vi "Execute.vi"(5 "SleepTerminalArray":refnum<vi>, 6 "ExeRef":refnum<vi>, 7 "ActiveTerminalArray":refnum<vi>, 8 "error in (no error)":errorcluster, 9 "Json_In":string, 10 "VariableRef":T2, 11 "Info":T1) -> (0 "Error Out":errorcluster, 1 "NumResultArray":dbl[](array[numeric]), 2 "StrResultArray":string[](array[string]), 3 "StrResult":string, 4 "NumResult":dbl)   [LabVIEW 2018, in "Array.lvlib"]
uses:
  Array.lvlib
  <userlib>/_OpenG.lib/dictionary/dictionary.llb/Dictionary Object RefNum__ogtk.ctl
  <userlib>/_OpenG.lib/dictionary/dictionary.llb/Dictionary Object RefNum - Enum__ogtk.ctl
  <userlib>/_MGI/1D Array/MGI Average/MGI Average (DBL[]).vi
  <userlib>/_OpenG.lib/array/array.llb/Remove Duplicates from 1D Array (String)__ogtk.vi
  <vilib>/addons/_JKI.lib/Serialization/JSON/JKI JSON Serialization.lvlib
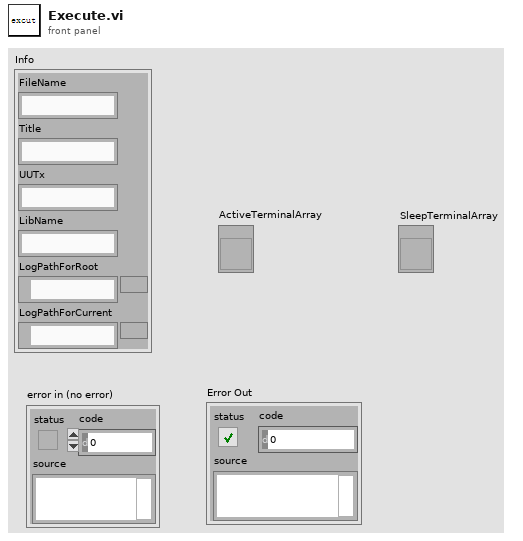
[diagram p1: front panel]
types:
  T1 = cluster{"FileName":string, "Title":string, "UUTx":string, "LibName":string, "LogPathForRoot":path, "LogPathForCurrent":path}
  T2 = typedef "Dictionary Object RefNum__ogtk.ctl" = refnum<k1>
  T3 = cluster{"ArraySize":cluster{"json":cluster{"Method":string, "ArrayVar":string}}, "IndexArray":cluster{"json":cluster{"Method":string, "ArrayVar":string, "Index":i32}}, "BuildArray":cluster{"json":cluster{"Method":string, "FirstElementVar":string, "SecondElementVar":string}}, "InsertIntoArray":cluster{"json":cluster{"Method":string, "ArrayVar":string, "Index":i32, "SubArrayVar":string}}, "DeleteFromArray":cluster{"json":cluster{"Method":string, "ArrayVar":string, "Index":i32, "Length":i32}}, "InitializeArray":cluster{"json":cluster{"Method":string, "ElementVar":string, "DimensionSize":i32}}, "ArraySubset":cluster{"json":cluster{"Method":string, "ArrayVar":string, "Index":i32, "Length":i32}}, "ArrayMax":cluster{"json":cluster{"Method":string, "ArrayVar":string}}, "ArrayMin":cluster{"json":cluster{"Method":string, "ArrayVar":string}}, "SearchArray":cluster{"json":cluster{"Method":string, "ArrayVar":string, "ElementVar":string, "StartIndex":i32}}, "ReplaceArraySubset":cluster{"json":cluster{"Method":string, "ArrayVar":string, "Index":i32, "SubArrayVar":string}}, "SortArray":cluster{"json":cluster{"Method":string, "ArrayVar":string}}, "ReverseArray":cluster{"json":cluster{"Method":string, "ArrayVar":string}}, "ArrayAverage":cluster{"json":cluster{"Method":string, "NumArrayVar":string, "IgnoreNaN":bool}}, "RemoveDuplicatesFromArray":cluster{"json":cluster{"Method":string, "ArrayVar":string}}, "ArrayToString":cluster{"json":cluster{"Method":string, "ArrayVar":string, "Delimiter":string}}}
  T4 = cluster{"json":cluster{"Method":string, "ArrayVar":string}}
  T5 = cluster{"json":cluster{"Method":string, "ArrayVar":string, "Index":i32}}
  T6 = cluster{"json":cluster{"Method":string, "FirstElementVar":string, "SecondElementVar":string}}
  T7 = cluster{"json":cluster{"Method":string, "ArrayVar":string, "Index":i32, "SubArrayVar":string}}
  T8 = cluster{"json":cluster{"Method":string, "ArrayVar":string, "Index":i32, "Length":i32}}
  T9 = cluster{"json":cluster{"Method":string, "ElementVar":string, "DimensionSize":i32}}
  T10 = cluster{"json":cluster{"Method":string, "ArrayVar":string, "ElementVar":string, "StartIndex":i32}}
  T11 = cluster{"json":cluster{"Method":string, "NumArrayVar":string, "IgnoreNaN":bool}}
  T12 = cluster{"json":cluster{"Method":string, "ArrayVar":string, "Delimiter":string}}
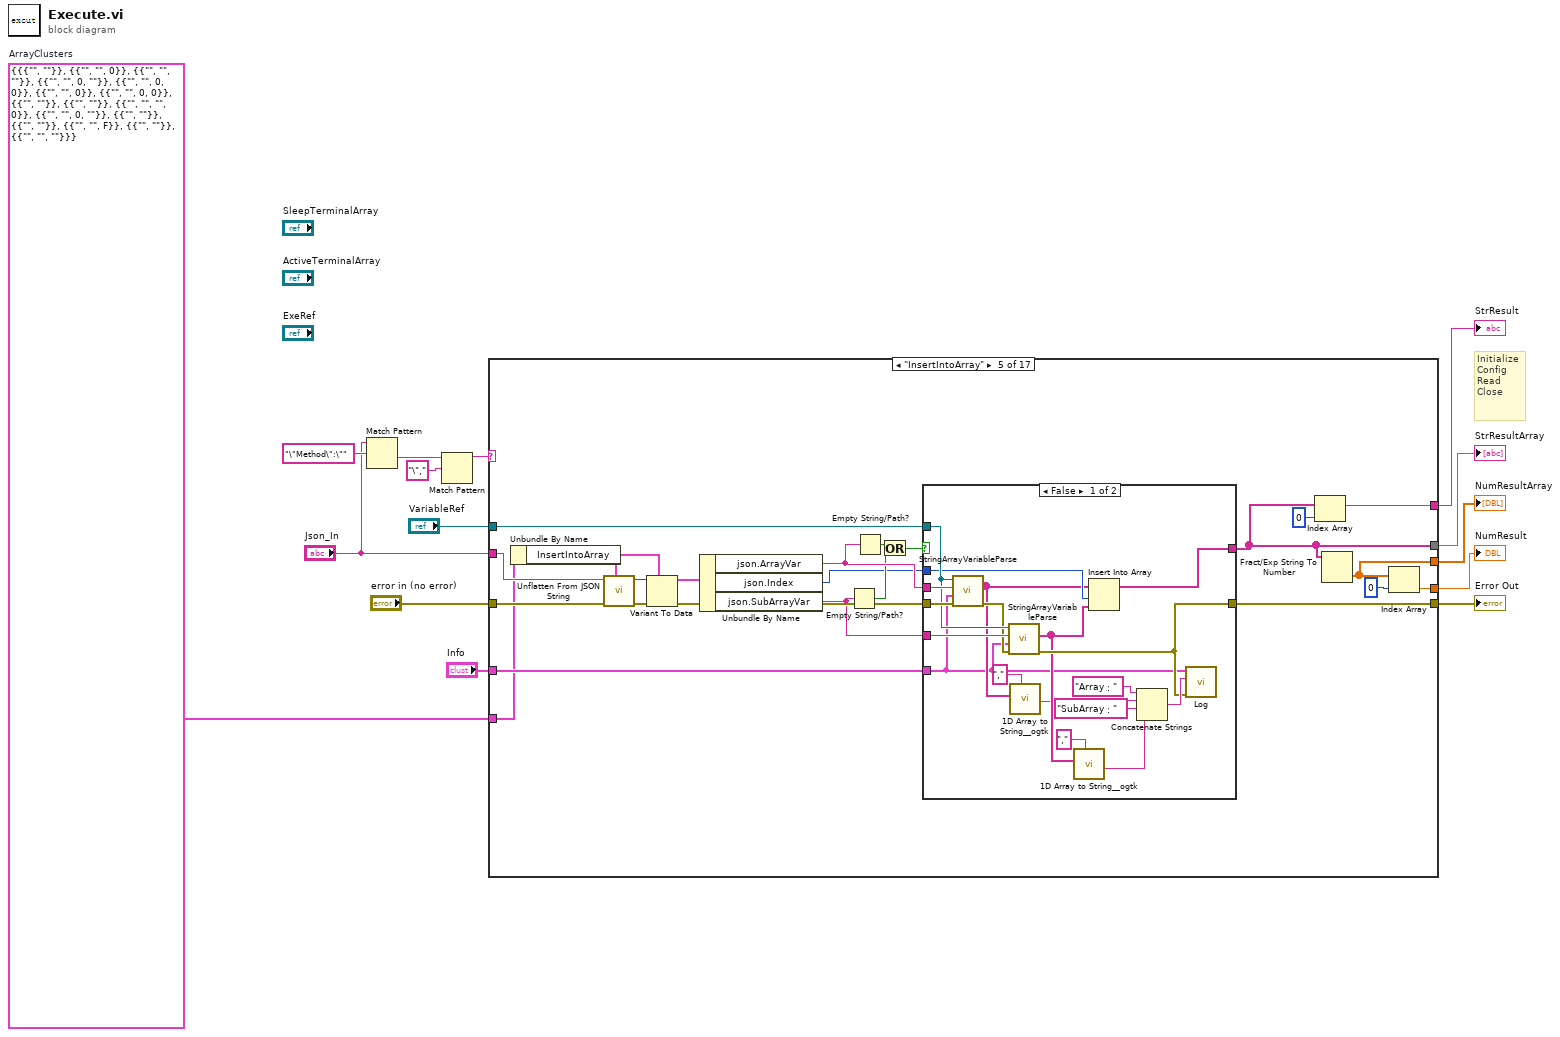
[diagram p0: block diagram]
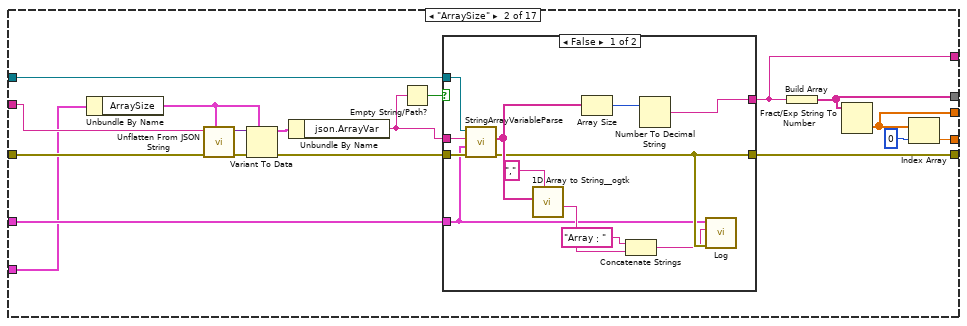
[diagram p3: hidden frame]
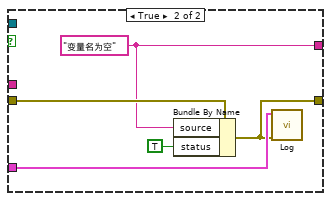
[diagram p4: hidden frame]
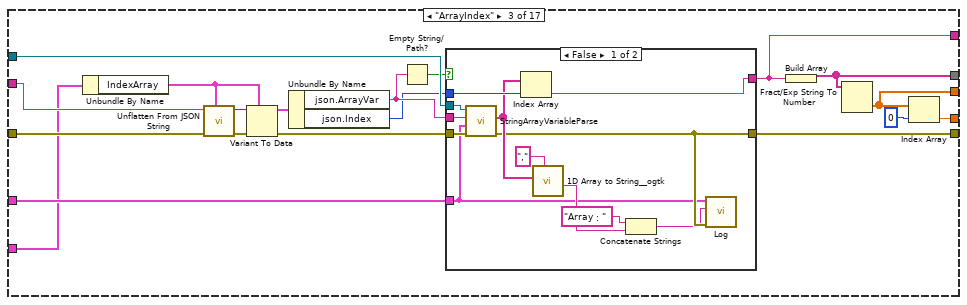
[diagram p5: hidden frame]
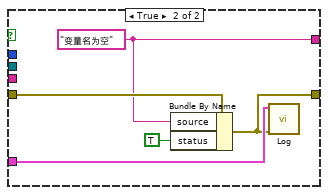
[diagram p6: hidden frame]
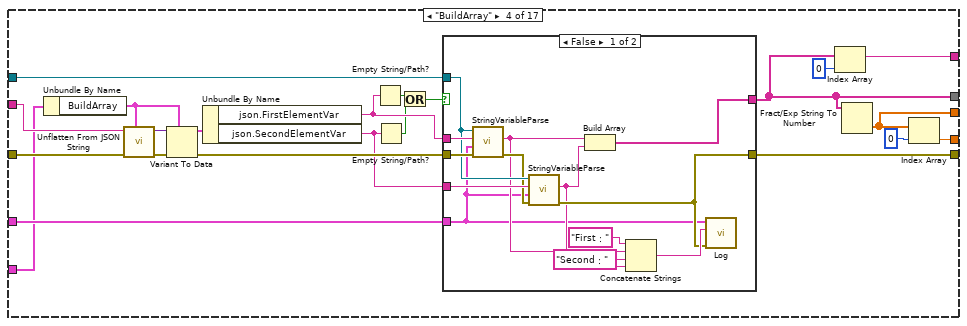
[diagram p7: hidden frame]
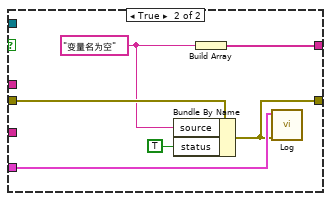
[diagram p8: hidden frame]
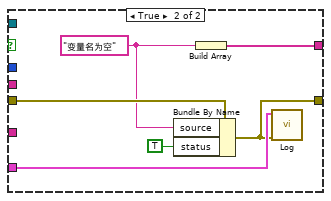
[diagram p9: hidden frame]
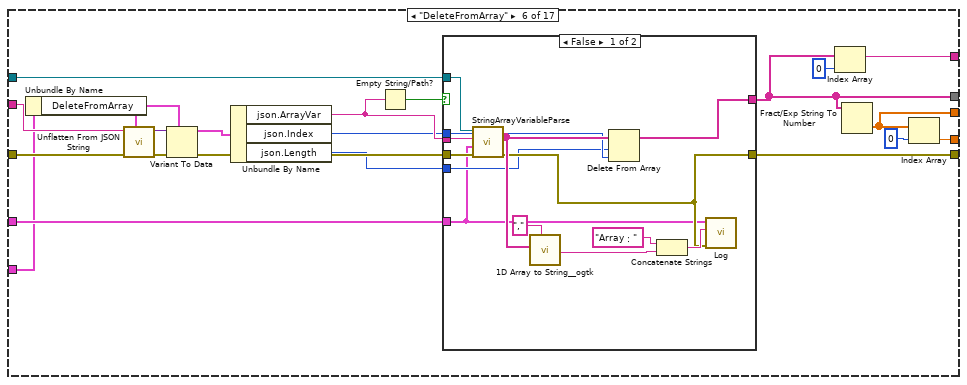
[diagram p10: hidden frame]
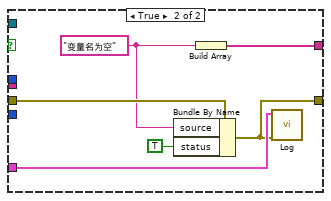
[diagram p11: hidden frame]
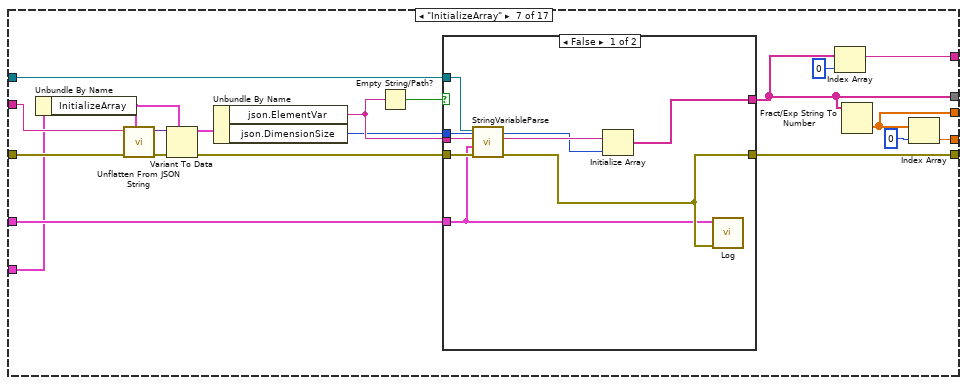
[diagram p12: hidden frame]
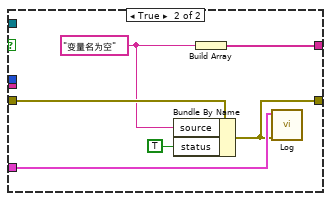
[diagram p13: hidden frame]
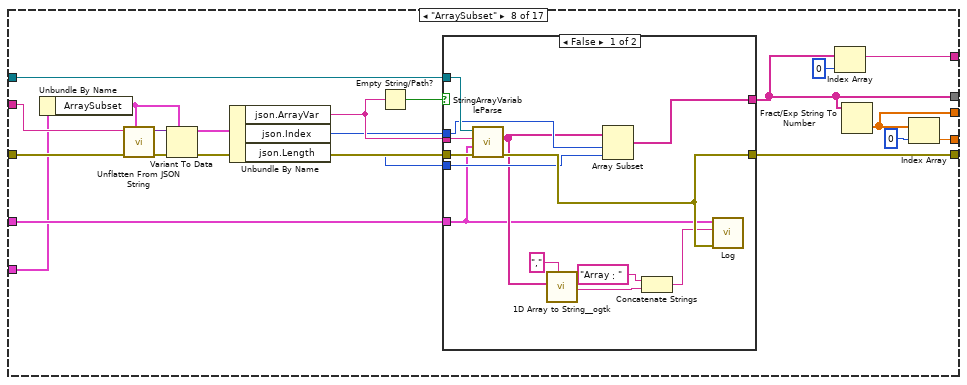
[diagram p14: hidden frame]
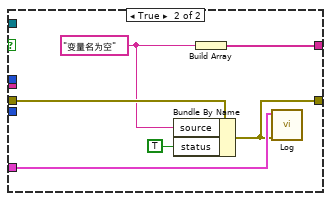
[diagram p15: hidden frame]
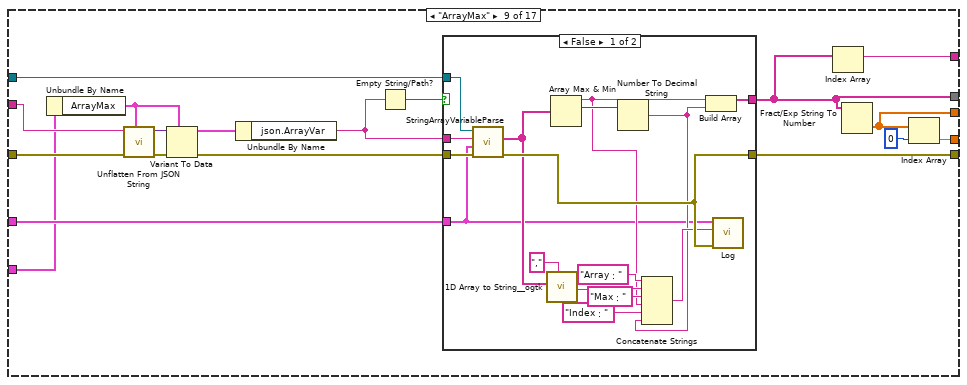
[diagram p16: hidden frame]
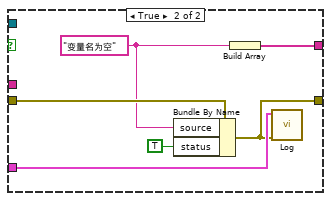
[diagram p17: hidden frame]
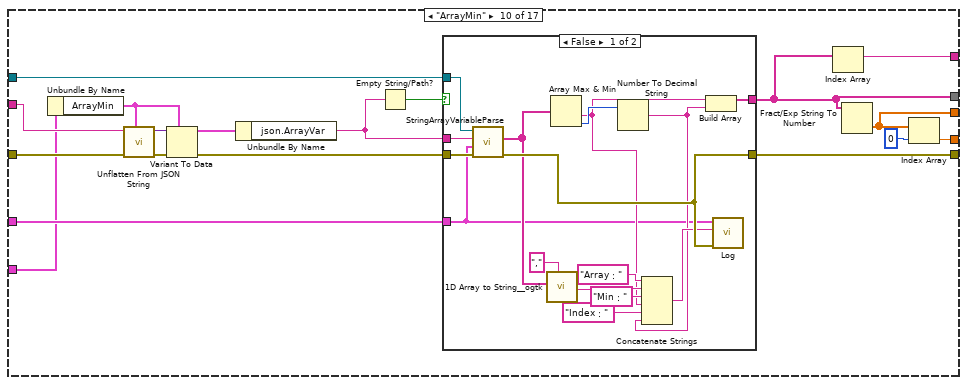
[diagram p18: hidden frame]
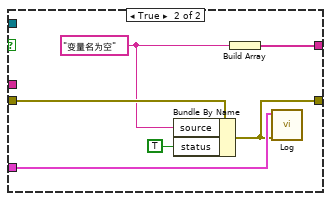
[diagram p19: hidden frame]
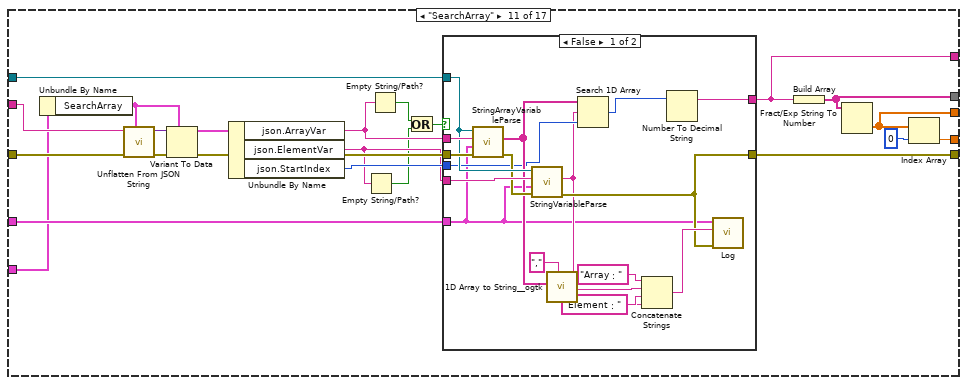
[diagram p20: hidden frame]
diagram:
  w1 = T3 {"ArraySize"={"json"={"Method"="", "ArrayVar"=""}}, "IndexArray"={"json"={"Method"="", "ArrayVar"="", "Index"=0}}, "BuildArray"={"json"={"Method"="", "FirstElementVar"="", "SecondElementVar"=""}}, "InsertIntoArray"={"json"={"Method"="", "ArrayVar"="", "Index"=0, "SubArrayVar"=""}}, "DeleteFromArray"={"json"={"Method"="", "ArrayVar"="", "Index"=0, "Length"=0}}, "InitializeArray"={"json"={"Method"="", "ElementVar"="", "DimensionSize"=0}}, "ArraySubset"={"json"={"Method"="", "ArrayVar"="", "Index"=0, "Length"=0}}, "ArrayMax"={"json"={"Method"="", "ArrayVar"=""}}, "ArrayMin"={"json"={"Method"="", "ArrayVar"=""}}, "SearchArray"={"json"={"Method"="", "ArrayVar"="", "ElementVar"="", "StartIndex"=0}}, "ReplaceArraySubset"={"json"={"Method"="", "ArrayVar"="", "Index"=0, "SubArrayVar"=""}}, "SortArray"={"json"={"Method"="", "ArrayVar"=""}}, "ReverseArray"={"json"={"Method"="", "ArrayVar"=""}}, "ArrayAverage"={"json"={"Method"="", "NumArrayVar"="", "IgnoreNaN"=FALSE}}, "RemoveDuplicatesFromArray"={"json"={"Method"="", "ArrayVar"=""}}, "ArrayToString"={"json"={"Method"="", "ArrayVar"="", "Delimiter"=""}}}  # ArrayClusters
  # "Initialize\nConfig\nRead\nClose"
  n1 = Match Pattern(string="Json_In", regular expression="\"Method\":\"") -> (after substring=w4:string)  [unwired: 1 in, 3 out]
  n2 = Match Pattern(string=w4, regular expression="\",") -> (before substring=w2:string)  [unwired: 1 in, 3 out]
  n3 = case shown="\"InsertIntoArray\"" w2 {
    tunnel: "Json_In" -> [_ w30 w66 w105 w147 w192 w231 w266 w303 w343 w387 w432 w475 w511 w547 w584 w620]
    tunnel: [w15 w25 w61 w100 w142 w188 w227 w262 w299 w339 w383 w428 w471 w507 w543 w580 w616] -> w14
    tunnel: "error in (no error)" -> [w15 w29 w65 w104 w146 w191 w230 w265 w302 w342 w386 w431 w474 w510 w546 w583 w619]
    tunnel: [_ w17 w52 w89 w132 w180 w219 w254 w289 w329 w370 w417 w461 w497 w533 w571 w606] -> w12
    tunnel: "VariableRef" -> [_ w27 w63 w102 w144 w189 w228 w263 w300 w340 w384 w429 w472 w508 w544 w581 w617]
    tunnel: [_ w16 w51 w87 w130 w178 w217 w252 w290 w330 w369 w418 w462 w498 w532 w570 w605] -> w11
    tunnel: [_ w20 w55 w95 w137 w183 w222 w257 w294 w334 w378 w423 w466 w502 w538 w575 w611] -> w10
    tunnel: [_ w22 w57 w97 w139 w185 w224 w259 w296 w336 w380 w425 w468 w504 w540 w577 w613] -> w9
    tunnel: "Info" -> [_ w23 w58 w98 w140 w186 w225 w260 w297 w337 w381 w426 w469 w505 w541 w578 w614]
    tunnel: w1 -> [_ w19 w54 w94 w136 w182 w221 w256 w293 w333 w377 w422 w465 w501 w537 w574 w610]
    frame Default {
    }
    frame "ArraySize" {
      n4 = Unbundle By Name(w19) -> ("ArraySize"=w18:T4)
      n5 = call <vilib>:"Unflatten From JSON String.vi"("Type and Defaults"=w18, "error in (no error)"=w29, "JSON String"=w30) -> ("error out"=w32:errorcluster, "Variant"=w33:variant)  [unwired: 7 in]
      n6 = Variant To Data(error in=w32, type=w18, Variant=w33) -> (data=w31:T4, error out=w28:errorcluster)
      n7 = Unbundle By Name(w31) -> ("json.ArrayVar"=w24:string)
      n8 = Empty String/Path?(string/path=w24) -> (empty?=w26:bool)
      n9 = case shown="False" w26 {
        tunnel: w28 -> [w45 w50]
        tunnel: w27 -> [w43 _]
        tunnel: [w38 w46] -> w25
        tunnel: w24 -> [w44 _]
        tunnel: [w35 w48] -> w17
        tunnel: w23 -> [w34 w47]
        frame False {
          n10 = call "StringArrayVariableParse.vi"("error in"=w45, "Info"=w34, "in"=w44, "dictionary"=w43) -> ("error out"=w38:errorcluster, "ValueArray"=w42:string[])  [unwired: 3 in, 3 out]
          n11 = call <userlib>:"1D Array to String__ogtk.vi"("delimiter (Tab)"=",", "Array of Strings"=w42) -> ("delimited string"=w39:string)  [unwired: 9 in]
          n12 = Array Size(array=w42) -> (size(s)=w36:i32)
          n13 = Concatenate Strings("Array：" ("string"), w39) -> (w37:string)
          n14 = Number To Decimal String(number=w36) -> (decimal integer string=w35:string)  [unwired: 1 in]
          n15 = call "Log.vi"("error in"=w38, "LogIn"=w37, "Info"=w34) -> ()  [unwired: 9 in]
        }
        frame True {
          w48 = "变量名为空" ("source")
          n16 = Bundle By Name(cluster=w50, "source"=w48, "status"=TRUE) -> (w46:errorcluster)
          n17 = call "Log.vi"("error in"=w46, "Info"=w47) -> ()  [unwired: 10 in]
        }
      }
      n18 = Build Array(w17) -> (w16:string[])
      n19 = Fract/Exp String To Number(string=w16) -> (number=w22:dbl[])  [unwired: 3 in, 1 out]
      n20 = Index Array(array=w22, index=0) -> (element=w20:dbl)
    }
    frame "ArrayIndex" {
      n21 = Unbundle By Name(w54) -> ("IndexArray"=w53:T5)
      n22 = call <vilib>:"Unflatten From JSON String.vi"("Type and Defaults"=w53, "error in (no error)"=w65, "JSON String"=w66) -> ("error out"=w68:errorcluster, "Variant"=w69:variant)  [unwired: 7 in]
      n23 = Variant To Data(error in=w68, type=w53, Variant=w69) -> (data=w67:T5, error out=w64:errorcluster)
      n24 = Unbundle By Name(w67) -> ("json.ArrayVar"=w60:string, "json.Index"=w59:i32)
      n25 = Empty String/Path?(string/path=w60) -> (empty?=w62:bool)
      n26 = case shown="False" w62 {
        tunnel: w64 -> [w80 w86]
        tunnel: w63 -> [w78 _]
        tunnel: [w73 w82] -> w61
        tunnel: w60 -> [w79 _]
        tunnel: [w71 w84] -> w52
        tunnel: w59 -> [w81 _]
        tunnel: w58 -> [w70 w83]
        frame False {
          n27 = call "StringArrayVariableParse.vi"("error in"=w80, "Info"=w70, "in"=w79, "dictionary"=w78) -> ("error out"=w73:errorcluster, "ValueArray"=w77:string[])  [unwired: 3 in, 3 out]
          n28 = Index Array(array=w77, index=w81) -> (element=w71:string)
          n29 = call <userlib>:"1D Array to String__ogtk.vi"("delimiter (Tab)"=",", "Array of Strings"=w77) -> ("delimited string"=w74:string)  [unwired: 9 in]
          n30 = Concatenate Strings("Array：" ("string"), w74) -> (w72:string)
          n31 = call "Log.vi"("error in"=w73, "LogIn"=w72, "Info"=w70) -> ()  [unwired: 9 in]
        }
        frame True {
          w84 = "变量名为空" ("source")
          n32 = Bundle By Name(cluster=w86, "source"=w84, "status"=TRUE) -> (w82:errorcluster)
          n33 = call "Log.vi"("error in"=w82, "Info"=w83) -> ()  [unwired: 10 in]
        }
      }
      n34 = Build Array(w52) -> (w51:string[])
      n35 = Fract/Exp String To Number(string=w51) -> (number=w57:dbl[])  [unwired: 3 in, 1 out]
      n36 = Index Array(array=w57, index=0) -> (element=w55:dbl)
    }
    frame "BuildArray" {
      n37 = Unbundle By Name(w94) -> ("BuildArray"=w93:T6)
      n38 = call <vilib>:"Unflatten From JSON String.vi"("Type and Defaults"=w93, "error in (no error)"=w104, "JSON String"=w105) -> ("error out"=w107:errorcluster, "Variant"=w108:variant)  [unwired: 7 in]
      n39 = Variant To Data(error in=w107, type=w93, Variant=w108) -> (data=w106:T6, error out=w103:errorcluster)
      n40 = Unbundle By Name(w106) -> ("json.FirstElementVar"=w99:string, "json.SecondElementVar"=w90:string)
      n41 = Empty String/Path?(string/path=w99) -> (empty?=w101:bool)
      n42 = Empty String/Path?(string/path=w90) -> (empty?=w91:bool)
      n43 = Or(x=w101, y=w91) -> (x .or. y?=w92:bool)
      n44 = case shown="False" w92 {
        tunnel: w103 -> [w118 w127]
        tunnel: w102 -> [w117 _]
        tunnel: [w114 w123] -> w100
        tunnel: w99 -> [w119 _]
        tunnel: [w113 w122] -> w87
        tunnel: w98 -> [w109 w124]
        tunnel: w90 -> [w116 _]
        frame False {
          n45 = call "StringVariableParse.vi"("error in"=w118, "Info"=w109, "in"=w119, "dictionary"=w117) -> ("error out"=w115:errorcluster, "out"=w112:string)  [unwired: 5 in, 1 out]
          n46 = call "StringVariableParse.vi"("error in"=w115, "Info"=w109, "in"=w116, "dictionary"=w117) -> ("error out"=w114:errorcluster, "out"=w110:string)  [unwired: 5 in, 1 out]
          n47 = Build Array(w112, w110) -> (w113:string[])
          n48 = Concatenate Strings("First：" ("string"), w112, "Second：" ("string"), w110) -> (w120:string)
          n49 = call "Log.vi"("error in"=w114, "LogIn"=w120, "Info"=w109) -> ()  [unwired: 9 in]
        }
        frame True {
          w125 = "变量名为空" ("source")
          n50 = Bundle By Name(cluster=w127, "source"=w125, "status"=TRUE) -> (w123:errorcluster)
          n51 = Build Array(w125) -> (w122:string[])
          n52 = call "Log.vi"("error in"=w123, "Info"=w124) -> ()  [unwired: 10 in]
        }
      }
      n53 = Index Array(array=w87, index=0) -> (element=w89:string)
      n54 = Fract/Exp String To Number(string=w87) -> (number=w97:dbl[])  [unwired: 3 in, 1 out]
      n55 = Index Array(array=w97, index=0) -> (element=w95:dbl)
    }
    frame "InsertIntoArray" {
      n56 = Unbundle By Name(w136) -> ("InsertIntoArray"=w135:T7)
      n57 = call <vilib>:"Unflatten From JSON String.vi"("Type and Defaults"=w135, "error in (no error)"=w146, "JSON String"=w147) -> ("error out"=w149:errorcluster, "Variant"=w150:variant)  [unwired: 7 in]
      n58 = Variant To Data(error in=w149, type=w135, Variant=w150) -> (data=w148:T7, error out=w145:errorcluster)
      n59 = Unbundle By Name(w148) -> ("json.ArrayVar"=w141:string, "json.Index"=w128:i32, "json.SubArrayVar"=w129:string)
      n60 = Empty String/Path?(string/path=w129) -> (empty?=w133:bool)
      n61 = Empty String/Path?(string/path=w141) -> (empty?=w143:bool)
      n62 = Or(x=w143, y=w133) -> (x .or. y?=w134:bool)
      n63 = case shown="False" w134 {
        tunnel: w145 -> [w165 w174]
        tunnel: w144 -> [w164 _]
        tunnel: [w161 w170] -> w142
        tunnel: w141 -> [w166 _]
        tunnel: [w160 w169] -> w130
        tunnel: w140 -> [w151 w171]
        tunnel: w129 -> [w163 _]
        tunnel: w128 -> [w158 _]
        frame False {
          n64 = call "StringArrayVariableParse.vi"("error in"=w165, "Info"=w151, "in"=w166, "dictionary"=w164) -> ("error out"=w162:errorcluster, "ValueArray"=w155:string[])  [unwired: 3 in, 3 out]
          n65 = call "StringArrayVariableParse.vi"("error in"=w162, "Info"=w151, "in"=w163, "dictionary"=w164) -> ("error out"=w161:errorcluster, "ValueArray"=w154:string[])  [unwired: 3 in, 3 out]
          n66 = call <userlib>:"1D Array to String__ogtk.vi"("delimiter (Tab)"=",", "Array of Strings"=w155) -> ("delimited string"=w153:string)  [unwired: 9 in]
          n67 = call <userlib>:"1D Array to String__ogtk.vi"("delimiter (Tab)"=",", "Array of Strings"=w154) -> ("delimited string"=w152:string)  [unwired: 9 in]
          n68 = Insert Into Array(array=w155, index=w158, new element=w154) -> (w160:string[])
          n69 = Concatenate Strings("Array：" ("string"), w153, "SubArray：" ("string"), w152) -> (w167:string)
          n70 = call "Log.vi"("error in"=w161, "LogIn"=w167, "Info"=w151) -> ()  [unwired: 9 in]
        }
        frame True {
          w172 = "变量名为空" ("source")
          n71 = Bundle By Name(cluster=w174, "source"=w172, "status"=TRUE) -> (w170:errorcluster)
          n72 = Build Array(w172) -> (w169:string[])
          n73 = call "Log.vi"("error in"=w170, "Info"=w171) -> ()  [unwired: 10 in]
        }
      }
      n74 = Index Array(array=w130, index=0) -> (element=w132:string)
      n75 = Fract/Exp String To Number(string=w130) -> (number=w139:dbl[])  [unwired: 3 in, 1 out]
      n76 = Index Array(array=w139, index=0) -> (element=w137:dbl)
    }
    frame "DeleteFromArray" {
      n77 = Unbundle By Name(w182) -> ("DeleteFromArray"=w181:T8)
      n78 = call <vilib>:"Unflatten From JSON String.vi"("Type and Defaults"=w181, "error in (no error)"=w191, "JSON String"=w192) -> ("error out"=w194:errorcluster, "Variant"=w195:variant)  [unwired: 7 in]
      n79 = Variant To Data(error in=w194, type=w181, Variant=w195) -> (data=w193:T8, error out=w190:errorcluster)
      n80 = Unbundle By Name(w193) -> ("json.ArrayVar"=w187:string, "json.Index"=w176:i32, "json.Length"=w177:i32)
      n81 = Empty String/Path?(string/path=w187) -> (empty?=w175:bool)
      n82 = case shown="False" w175 {
        tunnel: w190 -> [w205 w214]
        tunnel: w189 -> [w204 _]
        tunnel: [w199 w210] -> w188
        tunnel: w187 -> [w206 _]
        tunnel: [w203 w209] -> w178
        tunnel: w186 -> [w196 w211]
        tunnel: w177 -> [w197 _]
        tunnel: w176 -> [w198 _]
        frame False {
          n83 = call "StringArrayVariableParse.vi"("error in"=w205, "Info"=w196, "in"=w206, "dictionary"=w204) -> ("error out"=w199:errorcluster, "ValueArray"=w201:string[])  [unwired: 3 in, 3 out]
          n84 = call <userlib>:"1D Array to String__ogtk.vi"("delimiter (Tab)"=",", "Array of Strings"=w201) -> ("delimited string"=w200:string)  [unwired: 9 in]
          n85 = Delete From Array(array=w201, length=w197, index=w198) -> (array with subset deleted=w203:string[])  [unwired: 1 out]
          n86 = Concatenate Strings("Array：" ("string"), w200) -> (w207:string)
          n87 = call "Log.vi"("error in"=w199, "LogIn"=w207, "Info"=w196) -> ()  [unwired: 9 in]
        }
        frame True {
          w212 = "变量名为空" ("source")
          n88 = Bundle By Name(cluster=w214, "source"=w212, "status"=TRUE) -> (w210:errorcluster)
          n89 = Build Array(w212) -> (w209:string[])
          n90 = call "Log.vi"("error in"=w210, "Info"=w211) -> ()  [unwired: 10 in]
        }
      }
      n91 = Index Array(array=w178, index=0) -> (element=w180:string)
      n92 = Fract/Exp String To Number(string=w178) -> (number=w185:dbl[])  [unwired: 3 in, 1 out]
      n93 = Index Array(array=w185, index=0) -> (element=w183:dbl)
    }
    frame "InitializeArray" {
      n94 = Unbundle By Name(w221) -> ("InitializeArray"=w220:T9)
      n95 = call <vilib>:"Unflatten From JSON String.vi"("Type and Defaults"=w220, "error in (no error)"=w230, "JSON String"=w231) -> ("error out"=w233:errorcluster, "Variant"=w234:variant)  [unwired: 7 in]
      n96 = Variant To Data(error in=w233, type=w220, Variant=w234) -> (data=w232:T9, error out=w229:errorcluster)
      n97 = Unbundle By Name(w232) -> ("json.ElementVar"=w226:string, "json.DimensionSize"=w216:i32)
      n98 = Empty String/Path?(string/path=w226) -> (empty?=w215:bool)
      n99 = case shown="False" w215 {
        tunnel: w229 -> [w241 w248]
        tunnel: w228 -> [w240 _]
        tunnel: [w238 w244] -> w227
        tunnel: w226 -> [w242 _]
        tunnel: [w239 w243] -> w217
        tunnel: w225 -> [w235 w245]
        tunnel: w216 -> [w236 _]
        frame False {
          n100 = call "StringVariableParse.vi"("error in"=w241, "Info"=w235, "in"=w242, "dictionary"=w240) -> ("error out"=w238:errorcluster, "out"=w237:string)  [unwired: 5 in, 1 out]
          n101 = Initialize Array(w237, w236) -> (w239:string[])
          n102 = call "Log.vi"("error in"=w238, "Info"=w235) -> ()  [unwired: 10 in]
        }
        frame True {
          w246 = "变量名为空" ("source")
          n103 = Bundle By Name(cluster=w248, "source"=w246, "status"=TRUE) -> (w244:errorcluster)
          n104 = Build Array(w246) -> (w243:string[])
          n105 = call "Log.vi"("error in"=w244, "Info"=w245) -> ()  [unwired: 10 in]
        }
      }
      n106 = Index Array(array=w217, index=0) -> (element=w219:string)
      n107 = Fract/Exp String To Number(string=w217) -> (number=w224:dbl[])  [unwired: 3 in, 1 out]
      n108 = Index Array(array=w224, index=0) -> (element=w222:dbl)
    }
    frame "ArraySubset" {
      n109 = Unbundle By Name(w256) -> ("ArraySubset"=w255:T8)
      n110 = call <vilib>:"Unflatten From JSON String.vi"("Type and Defaults"=w255, "error in (no error)"=w265, "JSON String"=w266) -> ("error out"=w268:errorcluster, "Variant"=w269:variant)  [unwired: 7 in]
      n111 = Variant To Data(error in=w268, type=w255, Variant=w269) -> (data=w267:T8, error out=w264:errorcluster)
      n112 = Unbundle By Name(w267) -> ("json.ArrayVar"=w261:string, "json.Index"=w251:i32, "json.Length"=w249:i32)
      n113 = Empty String/Path?(string/path=w261) -> (empty?=w250:bool)
      n114 = case shown="False" w250 {
        tunnel: w264 -> [w281 w288]
        tunnel: w263 -> [w280 _]
        tunnel: [w278 w284] -> w262
        tunnel: w261 -> [w282 _]
        tunnel: [w279 w283] -> w252
        tunnel: w260 -> [w270 w285]
        tunnel: w251 -> [w277 _]
        tunnel: w249 -> [w276 _]
        frame False {
          n115 = call "StringArrayVariableParse.vi"("error in"=w281, "Info"=w270, "in"=w282, "dictionary"=w280) -> ("error out"=w278:errorcluster, "ValueArray"=w271:string[])  [unwired: 3 in, 3 out]
          n116 = call <userlib>:"1D Array to String__ogtk.vi"("delimiter (Tab)"=",", "Array of Strings"=w271) -> ("delimited string"=w274:string)  [unwired: 9 in]
          n117 = Array Subset(array=w271, index=w277, length=w276) -> (w279:string[])
          n118 = Concatenate Strings("Array：" ("string"), w274) -> (w272:string)
          n119 = call "Log.vi"("error in"=w278, "LogIn"=w272, "Info"=w270) -> ()  [unwired: 9 in]
        }
        frame True {
          w286 = "变量名为空" ("source")
          n120 = Bundle By Name(cluster=w288, "source"=w286, "status"=TRUE) -> (w284:errorcluster)
          n121 = Build Array(w286) -> (w283:string[])
          n122 = call "Log.vi"("error in"=w284, "Info"=w285) -> ()  [unwired: 10 in]
        }
      }
      n123 = Index Array(array=w252, index=0) -> (element=w254:string)
      n124 = Fract/Exp String To Number(string=w252) -> (number=w259:dbl[])  [unwired: 3 in, 1 out]
      n125 = Index Array(array=w259, index=0) -> (element=w257:dbl)
    }
    frame "ArrayMax" {
      n126 = Unbundle By Name(w293) -> ("ArrayMax"=w292:T4)
      n127 = call <vilib>:"Unflatten From JSON String.vi"("Type and Defaults"=w292, "error in (no error)"=w302, "JSON String"=w303) -> ("error out"=w305:errorcluster, "Variant"=w306:variant)  [unwired: 7 in]
      n128 = Variant To Data(error in=w305, type=w292, Variant=w306) -> (data=w304:T4, error out=w301:errorcluster)
      n129 = Unbundle By Name(w304) -> ("json.ArrayVar"=w298:string)
      n130 = Empty String/Path?(string/path=w298) -> (empty?=w291:bool)
      n131 = case shown="False" w291 {
        tunnel: w301 -> [w321 w328]
        tunnel: w300 -> [w320 _]
        tunnel: [w319 w325] -> w299
        tunnel: w298 -> [w322 _]
        tunnel: [w313 w323] -> w290
        tunnel: w297 -> [w307 w326]
        frame False {
          n132 = call "StringArrayVariableParse.vi"("error in"=w321, "Info"=w307, "in"=w322, "dictionary"=w320) -> ("error out"=w319:errorcluster, "ValueArray"=w314:string[])  [unwired: 3 in, 3 out]
          n133 = call <userlib>:"1D Array to String__ogtk.vi"("delimiter (Tab)"=",", "Array of Strings"=w314) -> ("delimited string"=w317:string)  [unwired: 9 in]
          n134 = Array Max & Min(array=w314) -> (max value=w310:string, max index (indices)=w312:i32)  [unwired: 2 out]
          n135 = Number To Decimal String(number=w312) -> (decimal integer string=w308:string)  [unwired: 1 in]
          n136 = Concatenate Strings("Array：" ("string"), w317, "Max：" ("string"), w310, "Index：" ("string"), w308) -> (w315:string)
          n137 = Build Array(w310, w308) -> (w313:string[])
          n138 = call "Log.vi"("error in"=w319, "LogIn"=w315, "Info"=w307) -> ()  [unwired: 9 in]
        }
        frame True {
          w324 = "变量名为空" ("source")
          n139 = Bundle By Name(cluster=w328, "source"=w324, "status"=TRUE) -> (w325:errorcluster)
          n140 = Build Array(w324) -> (w323:string[])
          n141 = call "Log.vi"("error in"=w325, "Info"=w326) -> ()  [unwired: 10 in]
        }
      }
      n142 = Index Array(array=w290) -> (element=w289:string)  [unwired: 1 in]
      n143 = Fract/Exp String To Number(string=w290) -> (number=w296:dbl[])  [unwired: 3 in, 1 out]
      n144 = Index Array(array=w296, index=0) -> (element=w294:dbl)
    }
    frame "ArrayMin" {
      n145 = Unbundle By Name(w333) -> ("ArrayMin"=w332:T4)
      n146 = call <vilib>:"Unflatten From JSON String.vi"("Type and Defaults"=w332, "error in (no error)"=w342, "JSON String"=w343) -> ("error out"=w345:errorcluster, "Variant"=w346:variant)  [unwired: 7 in]
      n147 = Variant To Data(error in=w345, type=w332, Variant=w346) -> (data=w344:T4, error out=w341:errorcluster)
      n148 = Unbundle By Name(w344) -> ("json.ArrayVar"=w338:string)
      n149 = Empty String/Path?(string/path=w338) -> (empty?=w331:bool)
      n150 = case shown="False" w331 {
        tunnel: w341 -> [w361 w368]
        tunnel: w340 -> [w360 _]
        tunnel: [w359 w365] -> w339
        tunnel: w338 -> [w362 _]
        tunnel: [w353 w363] -> w330
        tunnel: w337 -> [w347 w366]
        frame False {
          n151 = call "StringArrayVariableParse.vi"("error in"=w361, "Info"=w347, "in"=w362, "dictionary"=w360) -> ("error out"=w359:errorcluster, "ValueArray"=w354:string[])  [unwired: 3 in, 3 out]
          n152 = call <userlib>:"1D Array to String__ogtk.vi"("delimiter (Tab)"=",", "Array of Strings"=w354) -> ("delimited string"=w357:string)  [unwired: 9 in]
          n153 = Array Max & Min(array=w354) -> (min value=w348:string, min index (indices)=w349:i32)  [unwired: 2 out]
          n154 = Number To Decimal String(number=w349) -> (decimal integer string=w350:string)  [unwired: 1 in]
          n155 = Concatenate Strings("Array：" ("string"), w357, "Min：" ("string"), w348, "Index：" ("string"), w350) -> (w355:string)
          n156 = Build Array(w348, w350) -> (w353:string[])
          n157 = call "Log.vi"("error in"=w359, "LogIn"=w355, "Info"=w347) -> ()  [unwired: 9 in]
        }
        frame True {
          w364 = "变量名为空" ("source")
          n158 = Bundle By Name(cluster=w368, "source"=w364, "status"=TRUE) -> (w365:errorcluster)
          n159 = Build Array(w364) -> (w363:string[])
          n160 = call "Log.vi"("error in"=w365, "Info"=w366) -> ()  [unwired: 10 in]
        }
      }
      n161 = Index Array(array=w330) -> (element=w329:string)  [unwired: 1 in]
      n162 = Fract/Exp String To Number(string=w330) -> (number=w336:dbl[])  [unwired: 3 in, 1 out]
      n163 = Index Array(array=w336, index=0) -> (element=w334:dbl)
    }
    frame "SearchArray" {
      n164 = Unbundle By Name(w377) -> ("SearchArray"=w376:T10)
      n165 = call <vilib>:"Unflatten From JSON String.vi"("Type and Defaults"=w376, "error in (no error)"=w386, "JSON String"=w387) -> ("error out"=w389:errorcluster, "Variant"=w390:variant)  [unwired: 7 in]
      n166 = Variant To Data(error in=w389, type=w376, Variant=w390) -> (data=w388:T10, error out=w385:errorcluster)
      n167 = Unbundle By Name(w388) -> ("json.ArrayVar"=w382:string, "json.ElementVar"=w373:string, "json.StartIndex"=w374:i32)
      n168 = Empty String/Path?(string/path=w373) -> (empty?=w371:bool)
      n169 = Empty String/Path?(string/path=w382) -> (empty?=w375:bool)
      n170 = Or(x=w375, y=w371) -> (x .or. y?=w372:bool)
      n171 = case shown="False" w372 {
        tunnel: w385 -> [w406 w412]
        tunnel: w384 -> [w401 _]
        tunnel: [w398 w409] -> w383
        tunnel: w382 -> [w407 _]
        tunnel: [w394 w408] -> w370
        tunnel: w381 -> [w391 w410]
        tunnel: w373 -> [w400 _]
        tunnel: w374 -> [w396 _]
        frame False {
          n172 = call "StringArrayVariableParse.vi"("error in"=w406, "Info"=w391, "in"=w407, "dictionary"=w401) -> ("error out"=w399:errorcluster, "ValueArray"=w397:string[])  [unwired: 3 in, 3 out]
          n173 = call "StringVariableParse.vi"("error in"=w399, "Info"=w391, "in"=w400, "dictionary"=w401) -> ("error out"=w398:errorcluster, "out"=w392:string)  [unwired: 5 in, 1 out]
          n174 = call <userlib>:"1D Array to String__ogtk.vi"("delimiter (Tab)"=",", "Array of Strings"=w397) -> ("delimited string"=w404:string)  [unwired: 9 in]
          n175 = Search 1D Array(1D array=w397, element=w392, start index (0)=w396) -> (index of element=w395:i32)
          n176 = Concatenate Strings("Array：" ("string"), w404, "Element：" ("string"), w392) -> (w402:string)
          n177 = Number To Decimal String(number=w395) -> (decimal integer string=w394:string)  [unwired: 1 in]
          n178 = call "Log.vi"("error in"=w398, "LogIn"=w402, "Info"=w391) -> ()  [unwired: 9 in]
        }
        frame True {
          w408 = "变量名为空" ("source")
          n179 = Bundle By Name(cluster=w412, "source"=w408, "status"=TRUE) -> (w409:errorcluster)
          n180 = call "Log.vi"("error in"=w409, "Info"=w410) -> ()  [unwired: 10 in]
        }
      }
      n181 = Build Array(w370) -> (w369:string[])
      n182 = Fract/Exp String To Number(string=w369) -> (number=w380:dbl[])  [unwired: 3 in, 1 out]
      n183 = Index Array(array=w380, index=0) -> (element=w378:dbl)
    }
    frame "ReplaceArraySubset" {
      n184 = Unbundle By Name(w422) -> ("ReplaceArraySubset"=w421:T7)
      n185 = call <vilib>:"Unflatten From JSON String.vi"("Type and Defaults"=w421, "error in (no error)"=w431, "JSON String"=w432) -> ("error out"=w434:errorcluster, "Variant"=w435:variant)  [unwired: 7 in]
      n186 = Variant To Data(error in=w434, type=w421, Variant=w435) -> (data=w433:T7, error out=w430:errorcluster)
      n187 = Unbundle By Name(w433) -> ("json.ArrayVar"=w427:string, "json.Index"=w419:i32, "json.SubArrayVar"=w415:string)
      n188 = Empty String/Path?(string/path=w427) -> (empty?=w420:bool)
      n189 = Empty String/Path?(string/path=w415) -> (empty?=w413:bool)
      n190 = Or(x=w420, y=w413) -> (x .or. y?=w414:bool)
      n191 = case shown="False" w414 {
        tunnel: w430 -> [w452 w459]
        tunnel: w429 -> [w447 _]
        tunnel: [w445 w456] -> w428
        tunnel: w427 -> [w453 _]
        tunnel: [w440 w454] -> w418
        tunnel: w426 -> [w436 w457]
        tunnel: w415 -> [w443 _]
        tunnel: w419 -> [w441 _]
        frame False {
          n192 = call "StringArrayVariableParse.vi"("error in"=w452, "Info"=w436, "in"=w453, "dictionary"=w447) -> ("error out"=w446:errorcluster, "ValueArray"=w442:string[])  [unwired: 3 in, 3 out]
          n193 = call <userlib>:"1D Array to String__ogtk.vi"("delimiter (Tab)"=",", "Array of Strings"=w442) -> ("delimited string"=w450:string)  [unwired: 9 in]
          n194 = call "StringArrayVariableParse.vi"("error in"=w446, "Info"=w436, "in"=w443, "dictionary"=w447) -> ("error out"=w445:errorcluster, "ValueArray"=w437:string[])  [unwired: 3 in, 3 out]
          n195 = call <userlib>:"1D Array to String__ogtk.vi"("delimiter (Tab)"=",", "Array of Strings"=w437) -> ("delimited string"=w438:string)  [unwired: 9 in]
          n196 = Replace Array Subset(array=w442, new element=w437, index=w441) -> (w440:string[])
          n197 = Concatenate Strings("Array：" ("string"), w450, "SubArray：" ("string"), w438) -> (w448:string)
          n198 = call "Log.vi"("error in"=w445, "LogIn"=w448, "Info"=w436) -> ()  [unwired: 9 in]
        }
        frame True {
          w455 = "变量名为空" ("source")
          n199 = Bundle By Name(cluster=w459, "source"=w455, "status"=TRUE) -> (w456:errorcluster)
          n200 = Build Array(w455) -> (w454:string[])
          n201 = call "Log.vi"("error in"=w456, "Info"=w457) -> ()  [unwired: 10 in]
        }
      }
      n202 = Index Array(array=w418, index=0) -> (element=w417:string)
      n203 = Fract/Exp String To Number(string=w418) -> (number=w425:dbl[])  [unwired: 3 in, 1 out]
      n204 = Index Array(array=w425, index=0) -> (element=w423:dbl)
    }
    frame "SortArray" {
      n205 = Unbundle By Name(w465) -> ("SortArray"=w464:T4)
      n206 = call <vilib>:"Unflatten From JSON String.vi"("Type and Defaults"=w464, "error in (no error)"=w474, "JSON String"=w475) -> ("error out"=w477:errorcluster, "Variant"=w478:variant)  [unwired: 7 in]
      n207 = Variant To Data(error in=w477, type=w464, Variant=w478) -> (data=w476:T4, error out=w473:errorcluster)
      n208 = Unbundle By Name(w476) -> ("json.ArrayVar"=w470:string)
      n209 = Empty String/Path?(string/path=w470) -> (empty?=w463:bool)
      n210 = case shown="False" w463 {
        tunnel: w473 -> [w488 w495]
        tunnel: w472 -> [w483 _]
        tunnel: [w480 w492] -> w471
        tunnel: w470 -> [w489 _]
        tunnel: [w481 w490] -> w462
        tunnel: w469 -> [w479 w493]
        frame False {
          n211 = call "StringArrayVariableParse.vi"("error in"=w488, "Info"=w479, "in"=w489, "dictionary"=w483) -> ("error out"=w480:errorcluster, "ValueArray"=w482:string[])  [unwired: 3 in, 3 out]
          n212 = call <userlib>:"1D Array to String__ogtk.vi"("delimiter (Tab)"=",", "Array of Strings"=w482) -> ("delimited string"=w486:string)  [unwired: 9 in]
          n213 = Sort 1D Array(array=w482) -> (sorted array=w481:string[])
          n214 = Concatenate Strings("Array：" ("string"), w486) -> (w484:string)
          n215 = call "Log.vi"("error in"=w480, "LogIn"=w484, "Info"=w479) -> ()  [unwired: 9 in]
        }
        frame True {
          w491 = "变量名为空" ("source")
          n216 = Bundle By Name(cluster=w495, "source"=w491, "status"=TRUE) -> (w492:errorcluster)
          n217 = Build Array(w491) -> (w490:string[])
          n218 = call "Log.vi"("error in"=w492, "Info"=w493) -> ()  [unwired: 10 in]
        }
      }
      n219 = Index Array(array=w462, index=0) -> (element=w461:string)
      n220 = Fract/Exp String To Number(string=w462) -> (number=w468:dbl[])  [unwired: 3 in, 1 out]
      n221 = Index Array(array=w468, index=0) -> (element=w466:dbl)
    }
    frame "ReverseArray" {
      n222 = Unbundle By Name(w501) -> ("ReverseArray"=w500:T4)
      n223 = call <vilib>:"Unflatten From JSON String.vi"("Type and Defaults"=w500, "error in (no error)"=w510, "JSON String"=w511) -> ("error out"=w513:errorcluster, "Variant"=w514:variant)  [unwired: 7 in]
      n224 = Variant To Data(error in=w513, type=w500, Variant=w514) -> (data=w512:T4, error out=w509:errorcluster)
      n225 = Unbundle By Name(w512) -> ("json.ArrayVar"=w506:string)
      n226 = Empty String/Path?(string/path=w506) -> (empty?=w499:bool)
      n227 = case shown="False" w499 {
        tunnel: w509 -> [w524 w531]
        tunnel: w508 -> [w519 _]
        tunnel: [w516 w528] -> w507
        tunnel: w506 -> [w525 _]
        tunnel: [w517 w526] -> w498
        tunnel: w505 -> [w515 w529]
        frame False {
          n228 = call "StringArrayVariableParse.vi"("error in"=w524, "Info"=w515, "in"=w525, "dictionary"=w519) -> ("error out"=w516:errorcluster, "ValueArray"=w518:string[])  [unwired: 3 in, 3 out]
          n229 = call <userlib>:"1D Array to String__ogtk.vi"("delimiter (Tab)"=",", "Array of Strings"=w518) -> ("delimited string"=w522:string)  [unwired: 9 in]
          n230 = Reverse 1D Array(array=w518) -> (reversed array=w517:string[])
          n231 = Concatenate Strings("Array：" ("string"), w522) -> (w520:string)
          n232 = call "Log.vi"("error in"=w516, "LogIn"=w520, "Info"=w515) -> ()  [unwired: 9 in]
        }
        frame True {
          w527 = "变量名为空" ("source")
          n233 = Bundle By Name(cluster=w531, "source"=w527, "status"=TRUE) -> (w528:errorcluster)
          n234 = Build Array(w527) -> (w526:string[])
          n235 = call "Log.vi"("error in"=w528, "Info"=w529) -> ()  [unwired: 10 in]
        }
      }
      n236 = Index Array(array=w498, index=0) -> (element=w497:string)
      n237 = Fract/Exp String To Number(string=w498) -> (number=w504:dbl[])  [unwired: 3 in, 1 out]
      n238 = Index Array(array=w504, index=0) -> (element=w502:dbl)
    }
    frame "ArrayAverage" {
      n239 = Unbundle By Name(w537) -> ("ArrayAverage"=w536:T11)
      n240 = call <vilib>:"Unflatten From JSON String.vi"("Type and Defaults"=w536, "error in (no error)"=w546, "JSON String"=w547) -> ("error out"=w549:errorcluster, "Variant"=w550:variant)  [unwired: 7 in]
      n241 = Variant To Data(error in=w549, type=w536, Variant=w550) -> (data=w548:T11, error out=w545:errorcluster)
      n242 = Unbundle By Name(w548) -> ("json.NumArrayVar"=w542:string, "json.IgnoreNaN"=w534:bool)
      n243 = Empty String/Path?(string/path=w542) -> (empty?=w535:bool)
      n244 = case shown="False" w535 {
        tunnel: w545 -> [w563 w569]
        tunnel: w544 -> [w558 _]
        tunnel: [w557 w566] -> w543
        tunnel: w542 -> [w564 _]
        tunnel: [w552 w565] -> w533
        tunnel: w541 -> [w551 w567]
        tunnel: w534 -> [w554 _]
        frame False {
          n245 = call "StringArrayVariableParse.vi"("error in"=w563, "Info"=w551, "in"=w564, "dictionary"=w558) -> ("error out"=w557:errorcluster, "ValueArray"=w556:string[])  [unwired: 3 in, 3 out]
          n246 = call <userlib>:"1D Array to String__ogtk.vi"("delimiter (Tab)"=",", "Array of Strings"=w556) -> ("delimited string"=w561:string)  [unwired: 9 in]
          n247 = Fract/Exp String To Number(string=w556) -> (number=w555:dbl[])  [unwired: 3 in, 1 out]
          n248 = call-poly <userlib>:"MGI Average.vi"("Double[]"=w555, "Ignore NaN? (F)"=w554) -> ("Average"=w553:dbl)
          n249 = Concatenate Strings("Array：" ("string"), w561) -> (w559:string)
          n250 = Number To Fractional String(number=w553) -> (F-format string=w552:string)  [unwired: 3 in]
          n251 = call "Log.vi"("error in"=w557, "LogIn"=w559, "Info"=w551) -> ()  [unwired: 9 in]
        }
        frame True {
          w565 = "变量名为空" ("source")
          n252 = Bundle By Name(cluster=w569, "source"=w565, "status"=TRUE) -> (w566:errorcluster)
          n253 = call "Log.vi"("error in"=w566, "Info"=w567) -> ()  [unwired: 10 in]
        }
      }
      n254 = Build Array(w533) -> (w532:string[])
      n255 = Fract/Exp String To Number(string=w532) -> (number=w540:dbl[])  [unwired: 3 in, 1 out]
      n256 = Index Array(array=w540, index=0) -> (element=w538:dbl)
    }
    frame "RemoveDuplicatesFromArray" {
      n257 = Unbundle By Name(w574) -> ("RemoveDuplicatesFromArray"=w573:T4)
      n258 = call <vilib>:"Unflatten From JSON String.vi"("Type and Defaults"=w573, "error in (no error)"=w583, "JSON String"=w584) -> ("error out"=w586:errorcluster, "Variant"=w587:variant)  [unwired: 7 in]
      n259 = Variant To Data(error in=w586, type=w573, Variant=w587) -> (data=w585:T4, error out=w582:errorcluster)
      n260 = Unbundle By Name(w585) -> ("json.ArrayVar"=w579:string)
      n261 = Empty String/Path?(string/path=w579) -> (empty?=w572:bool)
      n262 = case shown="False" w572 {
        tunnel: w582 -> [w597 w604]
        tunnel: w581 -> [w592 _]
        tunnel: [w591 w601] -> w580
        tunnel: w579 -> [w598 _]
        tunnel: [w589 w599] -> w570
        tunnel: w578 -> [w588 w602]
        frame False {
          n263 = call "StringArrayVariableParse.vi"("error in"=w597, "Info"=w588, "in"=w598, "dictionary"=w592) -> ("error out"=w591:errorcluster, "ValueArray"=w590:string[])  [unwired: 3 in, 3 out]
          n264 = call <userlib>:"1D Array to String__ogtk.vi"("delimiter (Tab)"=",", "Array of Strings"=w590) -> ("delimited string"=w595:string)  [unwired: 9 in]
          n265 = call-poly <userlib>:"Remove Duplicates from 1D Array__ogtk.vi"("Input Array"=w590) -> ("Output Array"=w589:string[])  [unwired: 1 out]
          n266 = Concatenate Strings("Array：" ("string"), w595) -> (w593:string)
          n267 = call "Log.vi"("error in"=w591, "LogIn"=w593, "Info"=w588) -> ()  [unwired: 9 in]
        }
        frame True {
          w600 = "变量名为空" ("source")
          n268 = Bundle By Name(cluster=w604, "source"=w600, "status"=TRUE) -> (w601:errorcluster)
          n269 = Build Array(w600) -> (w599:string[])
          n270 = call "Log.vi"("error in"=w601, "Info"=w602) -> ()  [unwired: 10 in]
        }
      }
      n271 = Index Array(array=w570) -> (element=w571:string)  [unwired: 1 in]
      n272 = Fract/Exp String To Number(string=w570) -> (number=w577:dbl[])  [unwired: 3 in, 1 out]
      n273 = Index Array(array=w577, index=0) -> (element=w575:dbl)
    }
    frame "ArrayToString" {
      n274 = Unbundle By Name(w610) -> ("ArrayToString"=w609:T12)
      n275 = call <vilib>:"Unflatten From JSON String.vi"("Type and Defaults"=w609, "error in (no error)"=w619, "JSON String"=w620) -> ("error out"=w622:errorcluster, "Variant"=w623:variant)  [unwired: 7 in]
      n276 = Variant To Data(error in=w622, type=w609, Variant=w623) -> (data=w621:T12, error out=w618:errorcluster)
      n277 = Unbundle By Name(w621) -> ("json.ArrayVar"=w615:string, "json.Delimiter"=w607:string)
      n278 = Empty String/Path?(string/path=w615) -> (empty?=w608:bool)
      n279 = case shown="False" w608 {
        tunnel: w618 -> [w635 w646]
        tunnel: w617 -> [w630 _]
        tunnel: [w629 w643] -> w616
        tunnel: w615 -> [w636 _]
        tunnel: [w627 w642] -> w606
        tunnel: w614 -> [w624 w644]
        tunnel: w607 -> [w626 _]
        frame False {
          n280 = call "StringArrayVariableParse.vi"("error in"=w635, "Info"=w624, "in"=w636, "dictionary"=w630) -> ("error out"=w629:errorcluster, "ValueArray"=w628:string[])  [unwired: 3 in, 3 out]
          n281 = case shown="Default" w626 {
            selector: w626 -> [_ _ _ w640 _]
            tunnel: ["\r" "\n" "\r\n" w640 "\t"] -> w625
            frame "CarriageReturn" {
            }
            frame "LineFeed" {
            }
            frame "EndofLine" {
            }
            frame Default {
            }
            frame "Tab" {
            }
          }
          n282 = call <userlib>:"1D Array to String__ogtk.vi"("delimiter (Tab)"=",", "Array of Strings"=w628) -> ("delimited string"=w633:string)  [unwired: 9 in]
          n283 = call <userlib>:"1D Array to String__ogtk.vi"("delimiter (Tab)"=w625, "Array of Strings"=w628) -> ("delimited string"=w627:string)  [unwired: 9 in]
          n284 = Concatenate Strings("Array：" ("string"), w633) -> (w631:string)
          n285 = call "Log.vi"("error in"=w629, "LogIn"=w631, "Info"=w624) -> ()  [unwired: 9 in]
        }
        frame True {
          w642 = "变量名为空" ("source")
          n286 = Bundle By Name(cluster=w646, "source"=w642, "status"=TRUE) -> (w643:errorcluster)
          n287 = call "Log.vi"("error in"=w643, "Info"=w644) -> ()  [unwired: 10 in]
        }
      }
      n288 = Build Array(w606) -> (w605:string[])
      n289 = Fract/Exp String To Number(string=w605) -> (number=w613:dbl[])  [unwired: 3 in, 1 out]
      n290 = Index Array(array=w613, index=0) -> (element=w611:dbl)
    }
  }
  "StrResult" <- w12
  "Error Out" <- w14
  "StrResultArray" <- w11
  "NumResult" <- w10
  "NumResultArray" <- w9
